vi "StreamReceiveAcquisitionChA.vi"() -> ()   [LabVIEW 2018]
uses:
  <resource>/objmgr/ni.dex.rc
panel:
  in  "stop 2":bool
  out "error out 3":errorcluster
  out "error out 2":errorcluster
  out "error out":errorcluster
  in  "stop":bool
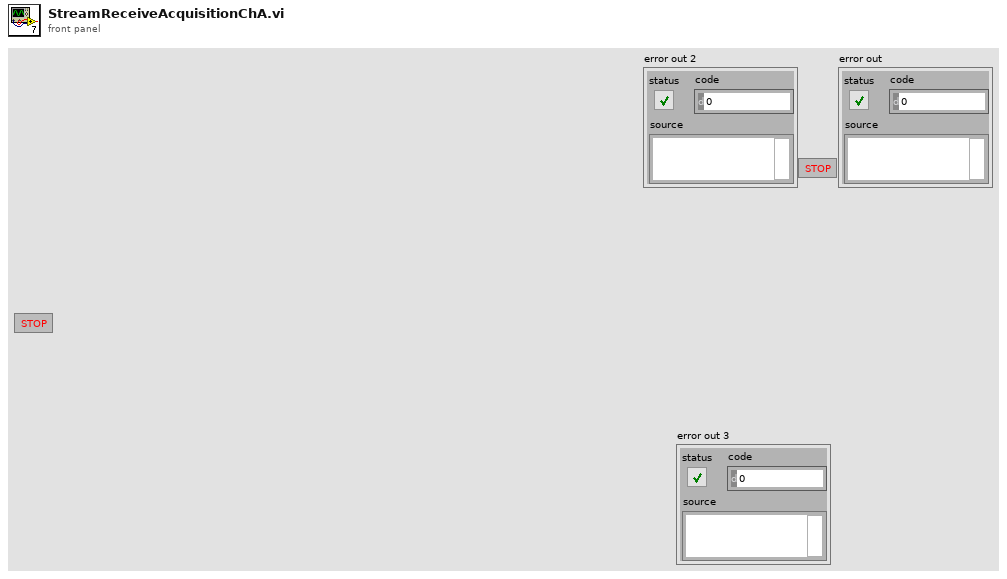
[diagram p1: front panel]
types:
  T1 = enum16{"Standard", "Buffered", "CRLF", "Immediate"}
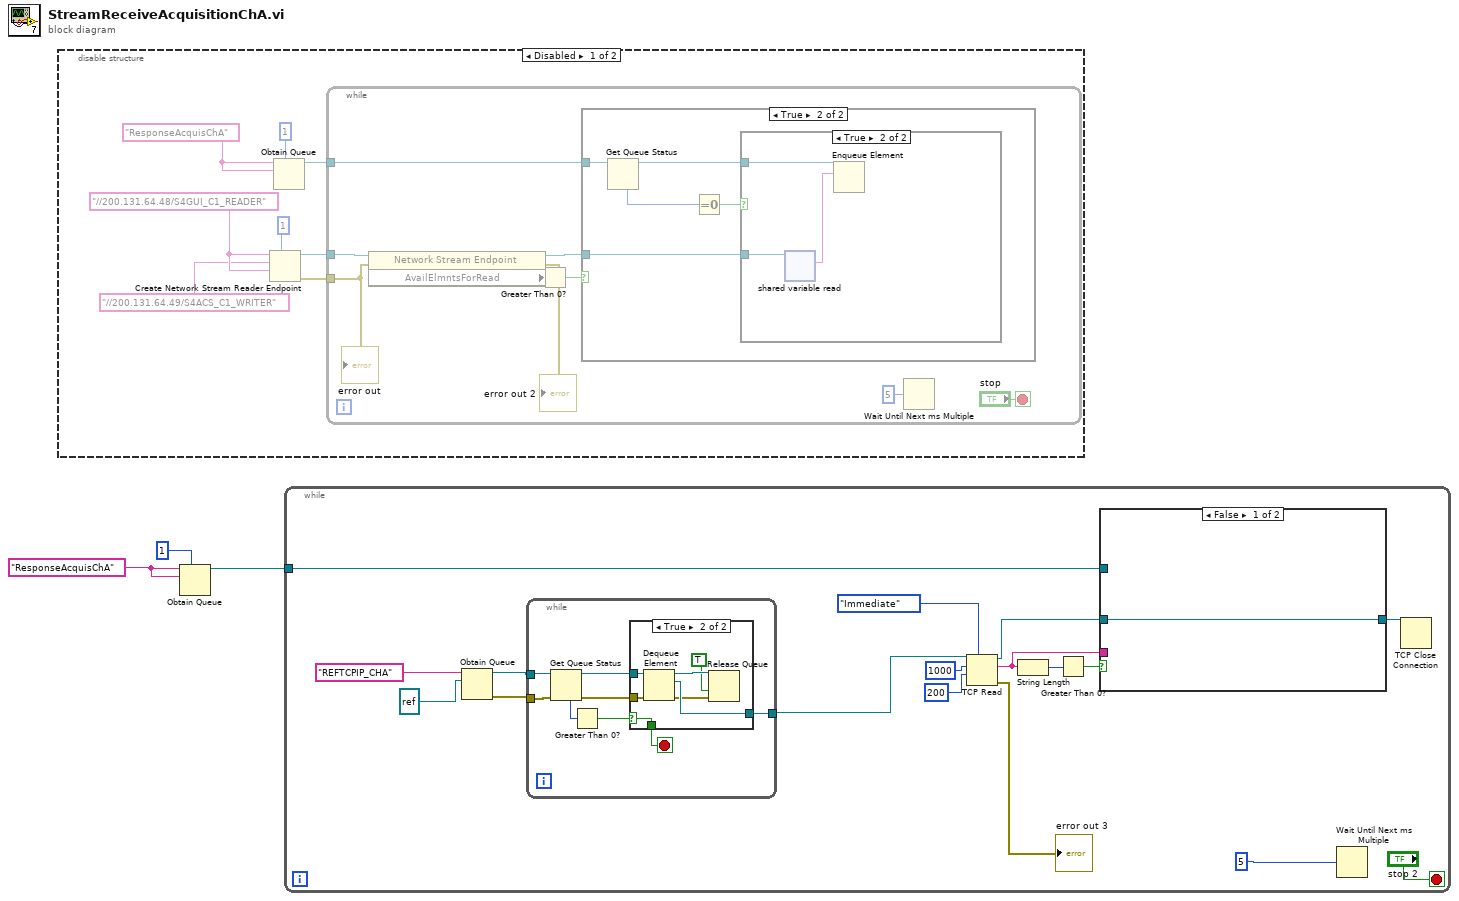
[diagram p0: block diagram]
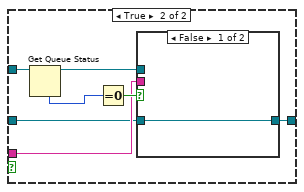
[diagram p6: hidden frame]
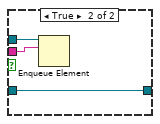
[diagram p7: hidden frame]
diagram:
  w1 = "ResponseAcquisChA"
  n1 = disable-structure shown="Disabled" {
    frame Disabled {
      w6 = "//200.131.64.48/S4GUI_C1_READER"
      w11 = "ResponseAcquisChA"
      n2 = Create Network Stream Reader Endpoint(7:1 ("reader buffer size"), 9:w6, 10:"//200.131.64.49/S4ACS_C1_WRITER", 11:w6) -> (0:w5:errorcluster, 3:w8:refnum<k21>)  [unwired: 3 in]
      n3 = Obtain Queue(max queue size (-1, unlimited)=1, name (unnamed)=w11, element data type=w11) -> (queue out=w10:refnum<queue>)  [unwired: 2 in, 2 out]
      n4 = while {
        tunnel: w10 -> [w19]
        tunnel: w8 -> [w18]
        tunnel: w5 -> [w12]
        stop <- "stop" stop-if-true
        n5 = property class="Network Stream Endpoint"(reference=w18, error in=w12) -> (reference out=w17:refnum<k21>, error out=→"error out 2":errorcluster, "AvailElmntsForRead"=w16:i32)
        n6 = Greater Than 0?(x=w16) -> (x > 0?=w15:bool)
        n7 = case shown="True" w15 {
          tunnel: w19 -> [_ w22]
          tunnel: w17 -> [_ w25]
          frame False {
          }
          frame True {
            n8 = Get Queue Status(queue=w22) -> (queue out=w21:refnum<queue>, # elements in queue=w24:i32)  [unwired: 2 in, 6 out]
            n9 = Equal To 0?(x=w24) -> (x = 0?=w23:bool)
            n10 = case shown="True" w23 {
              tunnel: w25 -> [_ w28]
              tunnel: w21 -> [_ w26]
              frame False {
              }
              frame True {
                n11 = shared-variable-read(w28) -> (w27:string)  [unwired: 2 in, 3 out]
                n12 = Enqueue Element(queue=w26, element=w27) -> ()  [unwired: 2 in, 3 out]
              }
            }
          }
        }
        n13 = Wait Until Next ms Multiple(millisecond multiple=u32 5) -> ()  [unwired: 1 out]
        "error out" <- w12
      }
    }
    frame Enabled {
    }
  }
  n14 = Obtain Queue(max queue size (-1, unlimited)=1, name (unnamed)=w1, element data type=w1) -> (queue out=w3:refnum<queue>)  [unwired: 2 in, 2 out]
  n15 = while {
    tunnel: w3 -> [w44]
    stop <- "stop 2" stop-if-true
    n16 = Obtain Queue(name (unnamed)="REFTCPIP_CHA", element data type=refnum<k5> refnum ("connection ID out")) -> (queue out=w31:refnum<queue>, error out=w30:errorcluster)  [unwired: 3 in, 1 out]
    n17 = while {
      tunnel: [w48] -> w34
      tunnel: w31 -> [w47]
      tunnel: w30 -> [w46]
      stop <- w49 stop-if-true
      n18 = Get Queue Status(queue=w47, error in (no error)=w46) -> (queue out=w53:refnum<queue>, error out=w52:errorcluster, # elements in queue=w50:i32)  [unwired: 1 in, 5 out]
      n19 = Greater Than 0?(x=w50) -> (x > 0?=w51:bool)
      n20 = case shown="True" w51 {
        selector: w51 -> [w54 w59]
        tunnel: w53 -> [_ w61]
        tunnel: w52 -> [_ w60]
        tunnel: [w54 w59] -> w49
        tunnel: [_ w58] -> w48
        frame False {
        }
        frame True {
          n21 = Dequeue Element(queue=w61, error in (no error)=w60) -> (queue out=w57:refnum<queue>, element=w58:refnum<k5>, error out=w56:errorcluster)  [unwired: 1 in, 1 out]
          n22 = Release Queue(queue=w57, force destroy? (F)=TRUE, error in (no error)=w56) -> ()  [unwired: 3 out]
        }
      }
    }
    n23 = TCP Read(connection ID=w34, bytes to read=1000, 7:T1."Immediate" ("mode (standard)"), 9:200 ("bytes to read")) -> (connection ID out=w35:refnum<k5>, data out=w40:string, error out=→"error out 3":errorcluster)  [unwired: 1 in]
    n24 = String Length(string=w40) -> (length=w42:i32)
    n25 = Greater Than 0?(x=w42) -> (x > 0?=w41:bool)
    n26 = case shown="False" w41 {
      tunnel: w44 -> [_ w67]
      tunnel: w40 -> [_ w65]
      tunnel: w35 -> [w62 w64]
      tunnel: [w62 w63] -> w29
      frame False {
      }
      frame True {
        n27 = Get Queue Status(queue=w67) -> (queue out=w66:refnum<queue>, # elements in queue=w69:i32)  [unwired: 2 in, 6 out]
        n28 = Equal To 0?(x=w69) -> (x = 0?=w68:bool)
        n29 = case shown="False" w68 {
          tunnel: w66 -> [_ w73]
          tunnel: w65 -> [_ w72]
          tunnel: w64 -> [w70 w71]
          tunnel: [w70 w71] -> w63
          frame False {
          }
          frame True {
            n30 = Enqueue Element(queue=w73, element=w72) -> ()  [unwired: 2 in, 3 out]
          }
        }
      }
    }
    n31 = Wait Until Next ms Multiple(millisecond multiple=u32 5) -> ()  [unwired: 1 out]
    n32 = TCP Close Connection(connection ID=w29) -> ()  [unwired: 2 in, 2 out]
  }
